vi "Write Raw CMD - Multiple Devices - Common Data.vi"(0 "Raw CMD":string, 11 "error in":errorcluster, 12 "FPGA":T1, 13 "Device Mask (All)":bool[](array[boolean])=[TRUE, TRUE, TRUE, TRUE, TRUE, TRUE], 14 "Log (T)":bool=TRUE) -> (15 "error out":errorcluster)   [LabVIEW 2017, in "Host SRL.lvlib"]
uses:
  Host SRL.lvlib
  Type Defs/WSVCAP SHL FPGA Enum.ctl
panel:
  # "DUT 01"
  # "DUT 02"
  # "DUT 03"
  # "DUT 04"
  # "DUT 05"
  # "DUT 06"
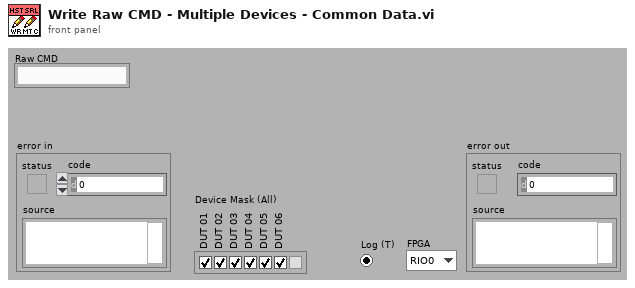
[diagram p1: front panel]
types:
  T1 = typedef "WSVCAP SHL FPGA Enum.ctl" = enum16{"RIO0", "RIO1"}
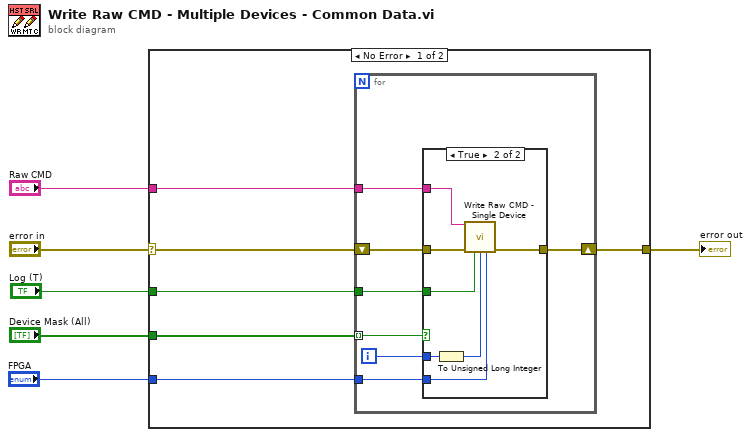
[diagram p0: block diagram]
diagram:
  n1 = case shown="No Error" "error in" {
    selector: "error in" -> [w12 _]
    tunnel: [w11 _] -> w6
    tunnel: "Raw CMD" -> [w7 _]
    tunnel: "Device Mask (All)" -> [w8 _]
    tunnel: "Log (T)" -> [w9 _]
    tunnel: "FPGA" -> [w10 _]
    frame No Error {
      n2 = for {
        tunnel: w7 -> [w18]
        shift-right: [w17] -> w11
        shift-left: w12 -> [w19]
        tunnel: w10 -> [w15]
        tunnel: w9 -> [w14]
        tunnel: w8 -> [w13] mode=indexing
        i -> [w16]
        n3 = case shown="True" w13 {
          tunnel: w19 -> [w20 w27]
          tunnel: w18 -> [_ w26]
          tunnel: [w20 w25] -> w17
          tunnel: w16 -> [_ w24]
          tunnel: w15 -> [_ w23]
          tunnel: w14 -> [_ w22]
          frame False {
          }
          frame True {
            n4 = To Unsigned Long Integer(number=w24) -> (unsigned 32bit integer=w21:u32)
            n5 = call "Write Raw CMD - Single Device.vi"("Data Out"=w26, "error in"=w27, "Log (T)"=w22, "Device Idx (0-5)"=w21, "FPGA"=w23) -> ("error out"=w25:errorcluster)  [unwired: 10 in]
          }
        }
      }
    }
    frame Error {
    }
  }
  "error out" <- w6
